vi "Project_Smart_System.vi"() -> ()   [LabVIEW 2020]
uses:
  <vilib>/LabVIEW Interface for Arduino/Type Defs/Analog Pin.ctl
  <vilib>/LabVIEW Interface for Arduino/Type Defs/Digital Pin.ctl
  <vilib>/LabVIEW Interface for Arduino/Type Defs/Board Type.ctl
  <vilib>/LabVIEW Interface for Arduino/LabVIEW Interface for Arduino.lvlib
panel:
  in  "Buzzer Pin":T1
  in  "Water Relay":T1
  in  "Fan Relay":T1
  in  "Smoke Input":T2
  in  "Temp Input":T2
  in  "Flame Input":T2
  out "Flame  Activate":bool
  in  "Flame Threshold":u8
  out "Temperature Activate":bool
  in  "Temperature Threshold":dbl
  out "Alarm Alert":bool
  in  "Smoke threshold":dbl
  out "Smoke Value":u8
  in  "Duration ms":u32=1
  in  "Frequency":u16=500 step=100
  in  "Tone DO Pin":u8=8
  in  "milliseconds to wait":u32
  in  "Stop":bool
  out "Temperature":dbl(slide) scale=0.0..100.0
  in  "Paired Resistance (Ohms)":dbl=10000.0
  in  "Units":enum16{"Celsius", "Fahrenheit", "Kelvin"}(ring)
  in  "VISA resource":refnum<visa-resource-name>
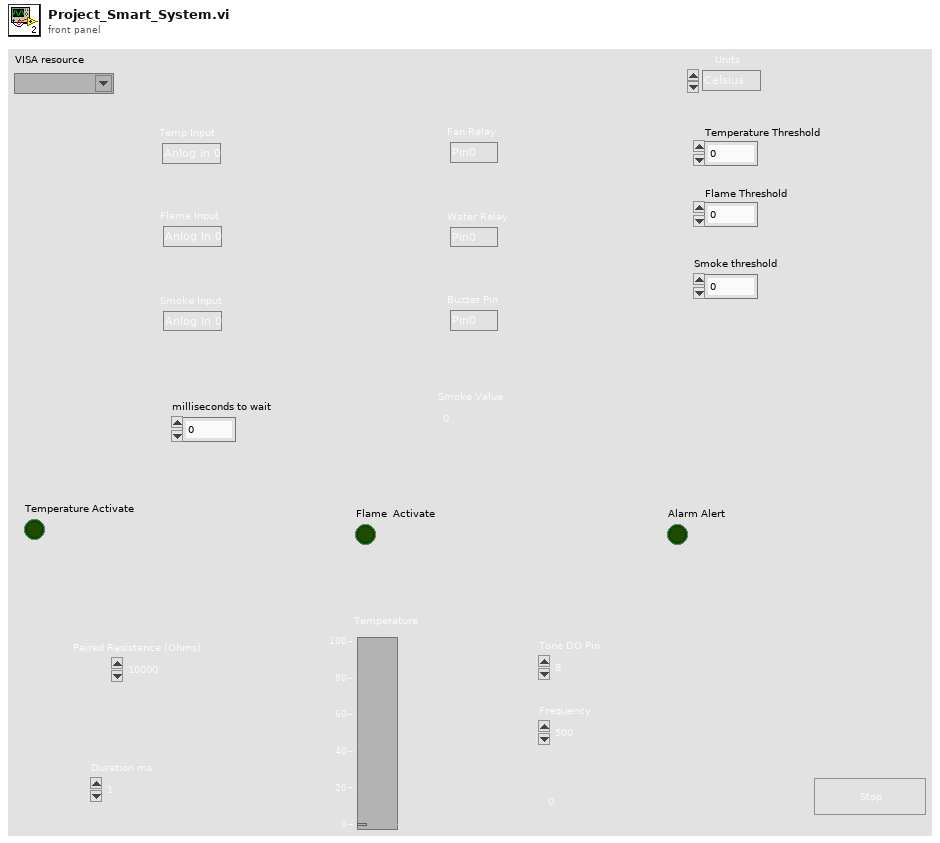
[diagram p1: front panel]
types:
  T1 = typedef "LabVIEW Interface for Arduino.lvlib/Digital Pin.ctl" = enum8{"Pin0", "Pin1", "Pin2", "Pin3", "Pin4", "Pin5", "Pin6", "Pin7", "Pin8", "Pin9", "Pin10", "Pin11", "Pin12", "Pin13"}
  T2 = typedef "LabVIEW Interface for Arduino.lvlib/Analog Pin.ctl" = enum8{"Anlog In 0", "Anlog In 1", "Anlog In 2", "Anlog In 3", "Anlog In 4", "Anlog In 5"}
  T3 = typedef "LabVIEW Interface for Arduino.lvlib/Board Type.ctl" = enum16{"Uno", "Dimuelanove w/Atmega 328", "Mega 2560"}
  T4 = typedef "LabVIEW Interface for Arduino.lvlib/Arduino Resource.ctl" = cluster{"VISA resource":refnum<visa-resource-name>, "Board Type":T3, "Connection Type":enum8{"USB / Serial"}, "Bytes Per Packet (15)":u8}
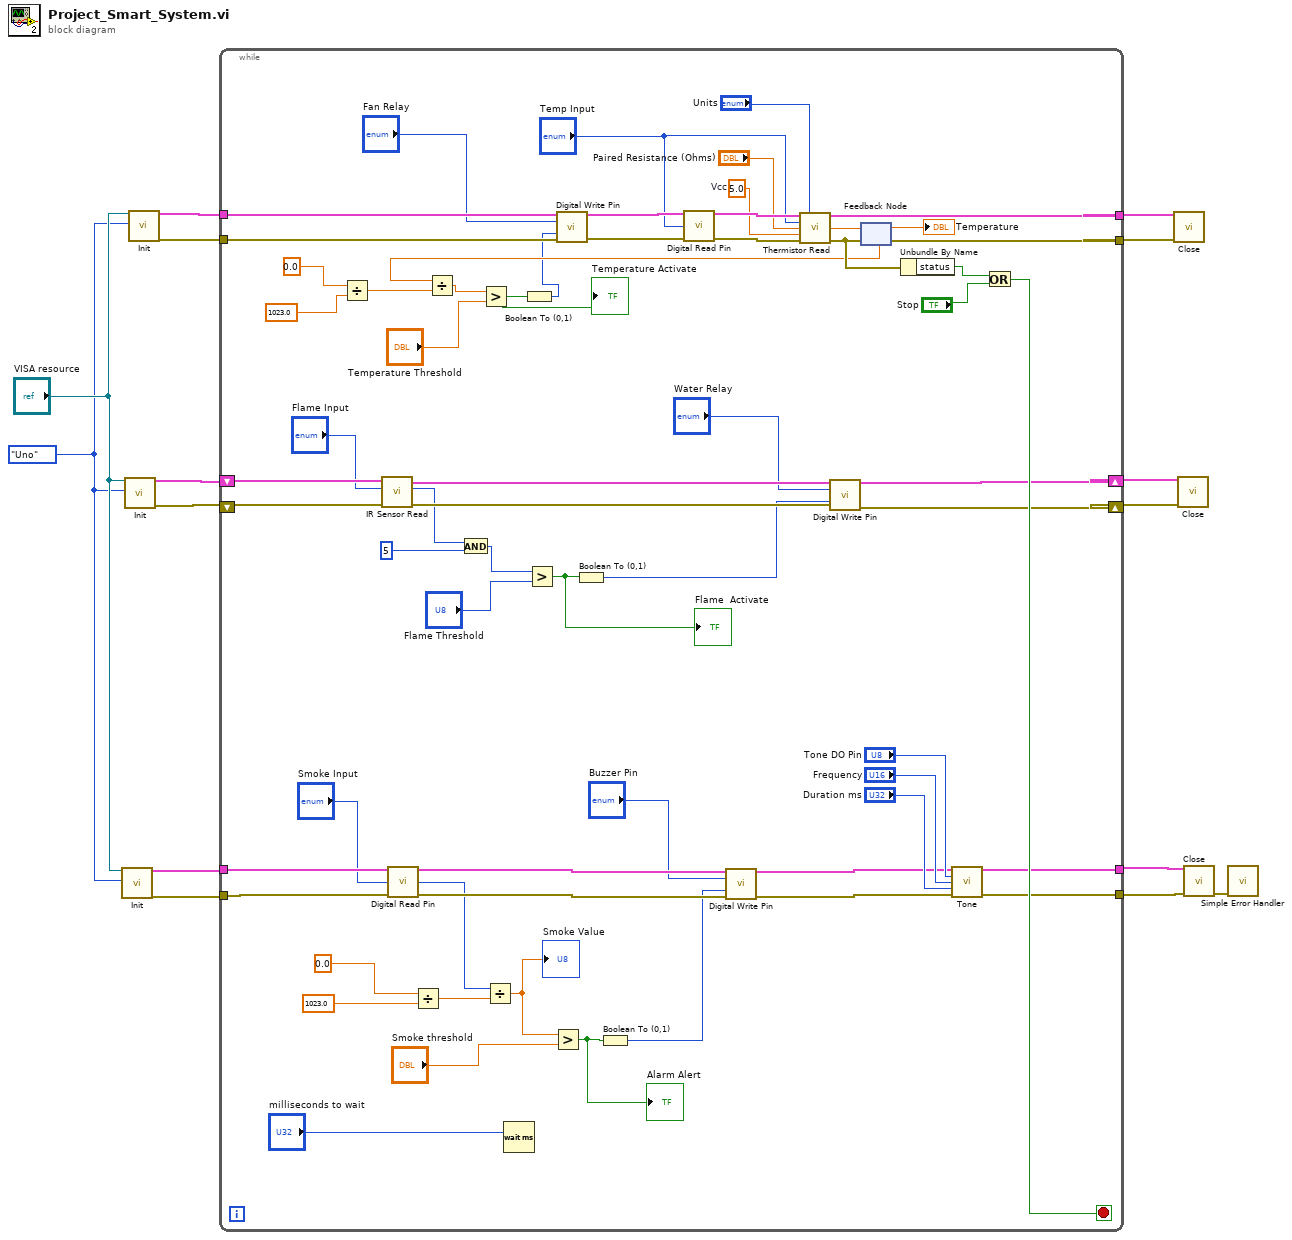
[diagram p0: block diagram]
diagram:
  w7 = Board_Type."Uno" ("Board Type (Uno)")
  n1 = call <vilib>:"Init.vi"("VISA resource"="VISA resource", "Board Type (Uno)"=w7) -> ("Arduino Resource"=w1:T4, "error out"=w11:errorcluster)  [unwired: 16 in]
  n2 = call <vilib>:"Init.vi"("VISA resource"="VISA resource", "Board Type (Uno)"=w7) -> ("Arduino Resource"=w15:T4, "error out"=w14:errorcluster)  [unwired: 16 in]
  n3 = call <vilib>:"Init.vi"("VISA resource"="VISA resource", "Board Type (Uno)"=w7) -> ("Arduino Resource"=w6:T4, "error out"=w3:errorcluster)  [unwired: 16 in]
  n4 = while {
    shift-right: [w30] -> w13
    shift-left: w15 -> [w33]
    shift-right: [w28] -> w12
    shift-left: w14 -> [w32]
    tunnel: w1 -> [w56]
    tunnel: w11 -> [w55]
    tunnel: [w60] -> w10
    tunnel: [w61] -> w9
    tunnel: w6 -> [w76]
    tunnel: [w70] -> w5
    tunnel: [w66] -> w4
    tunnel: w3 -> [w73]
    stop <- w63 stop-if-true
    w67 = 5.0  # Vcc
    n5 = Divide(x=0.0, y=1023.0) -> (x/y=w40:dbl)
    n6 = call <vilib>:"IR Sensor Read.vi"("error in"=w32, "Sensor Pin"="Flame Input", "Arduino Resource"=w33) -> ("error out"=w29:errorcluster, "MotionDetected"=w27:u8, "Arduino Resource"=w31:T4)  [unwired: 6 in]
    n7 = call <vilib>:"Digital Read Pin.vi"("Arduino Resource"=w56, "Digital I/O Pin (0)"="Smoke Input", "error in"=w55) -> ("Arduino Resource"=w54:T4, "Value"=w50:u8, "error out"=w53:errorcluster)  [unwired: 10 in]
    n8 = Divide(x=0.0, y=1023.0) -> (x/y=w49:dbl)
    n9 = And(x=w27, y=u8 5) -> (x .and. y?=w25:u8)
    n10 = Divide(x=w50, y=w49) -> (x/y=w46:dbl)
    "Smoke Value" <- w46
    n11 = Wait (ms)(milliseconds to wait="milliseconds to wait") -> ()  [unwired: 1 out]
    n12 = Greater?(x=w25, y="Flame Threshold") -> (0:w22:bool)
    "Flame  Activate" <- w22
    n13 = Greater?(x=w46, y="Smoke threshold") -> (0:w43:bool)
    "Alarm Alert" <- w43
    n14 = Boolean To (0,1)(Boolean=w22) -> (0, 1=w23:i16)
    n15 = Boolean To (0,1)(Boolean=w43) -> (0, 1=w44:i16)
    n16 = call <vilib>:"Digital Write Pin.vi"("Arduino Resource"=w54, "Digital I/O Pin (0)"="Buzzer Pin", "Value (0)"=w44, "error in"=w53) -> ("Arduino Resource"=w52:T4, "error out"=w51:errorcluster)  [unwired: 10 in]
    n17 = call <vilib>:"Digital Write Pin.vi"("Arduino Resource"=w31, "Digital I/O Pin (0)"="Water Relay", "Value (0)"=w23, "error in"=w29) -> ("Arduino Resource"=w30:T4, "error out"=w28:errorcluster)  [unwired: 10 in]
    n18 = feedback #1() -> (w41:dbl)  [unwired: 1 in]
    "Temperature" <- w41
    n19 = Divide(x=w41, y=w40) -> (x/y=w37:dbl)
    n20 = Greater?(x=w37, y="Temperature Threshold") -> (0:w34:bool)
    "Temperature Activate" <- w34
    n21 = Boolean To (0,1)(Boolean=w34) -> (0, 1=w35:i16)
    n22 = call <vilib>:"Digital Write Pin.vi"("Arduino Resource"=w76, "Digital I/O Pin (0)"="Fan Relay", "Value (0)"=w35, "error in"=w73) -> ("Arduino Resource"=w75:T4, "error out"=w74:errorcluster)  [unwired: 10 in]
    n23 = call <vilib>:"Digital Read Pin.vi"("Arduino Resource"=w75, "Digital I/O Pin (0)"="Temp Input", "error in"=w74) -> ("Arduino Resource"=w72:T4, "error out"=w71:errorcluster)  [unwired: 10 in, 1 out]
    n24 = call <vilib>:"Thermistor Read.vi"("Arduino Resource"=w72, "Units (C)"="Units", "Thermistor AI Pin (0)"="Temp Input", "Paired Resistance (10K Ohms)"="Paired Resistance (Ohms)", "Vcc (5 v)"=w67, "error in"=w71) -> ("Arduino Resource"=w70:T4, "Temperature"=w42:dbl, "error out"=w66:errorcluster)  [unwired: 7 in]
    n25 = feedback-in #1(w42) -> ()
    n26 = Unbundle By Name(w66) -> ("status"=w65:bool)
    n27 = call <vilib>:"Tone.vi"("Arduino Resource"=w52, "Tone DO Pin"="Tone DO Pin", "Frequency (0 Hz)"="Frequency", "Duration (1 ms)"="Duration ms", "error in"=w51) -> ("Arduino Resource"=w60:T4, "error out"=w61:errorcluster)  [unwired: 9 in]
    n28 = Or(x=w65, y="Stop") -> (x .or. y?=w63:bool)
  }
  n29 = call <vilib>:"Close.vi"("Arduino Resource"=w5, "error in"=w4) -> ()  [unwired: 13 in, 1 out]
  n30 = call <vilib>:"Close.vi"("Arduino Resource"=w13, "error in"=w12) -> ()  [unwired: 13 in, 1 out]
  n31 = call <vilib>:"Close.vi"("Arduino Resource"=w10, "error in"=w9) -> ("error out"=w2:errorcluster)  [unwired: 13 in]
  n32 = call <vilib>:"Simple Error Handler.vi"("error in (no error)"=w2) -> ()  [unwired: 4 in, 5 out]
